vi "Read Last Bus Load.vi"(8 "error in (no error)":errorcluster, 11 "GenBus_Load_Calculator in":refnum<class "CANBus_Load_Calculator.lvclass">) -> (0 "error out":errorcluster, 2 "Bus Load (%)":dbl, 3 "GenBus_Load_Calculator out":refnum<class "CANBus_Load_Calculator.lvclass">)   [LabVIEW 2018, in "NI-XNET Monitor Engine.lvlib" / "XNET-Bus-Load-Calculator.lvlib" / "CANBus_Load_Calculator.lvclass"]
uses:
  CANBus_Load_Calculator.lvclass
  CANBus_Load_Calculator.lvclass/CANBus_Load_Calculator.ctl
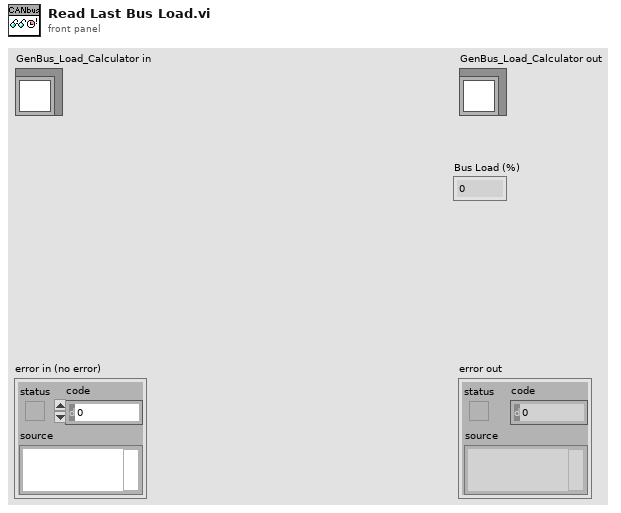
[diagram p1: front panel]
types:
  T1 = typedef "XNET-Bus-Load-Calculator.lvlib/CANBus_Load_Calculator.lvclass/FromCalculator_Data.ctl" = cluster{"Bus Load (%)":dbl}
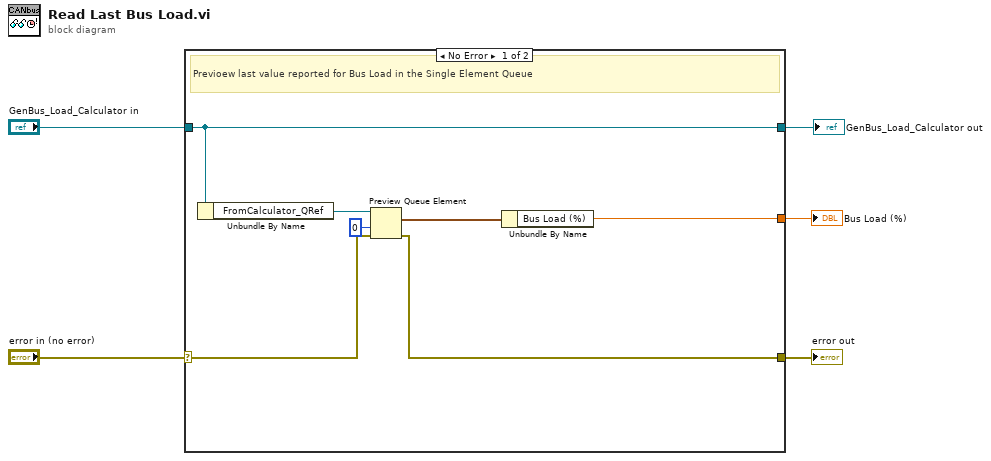
[diagram p0: block diagram]
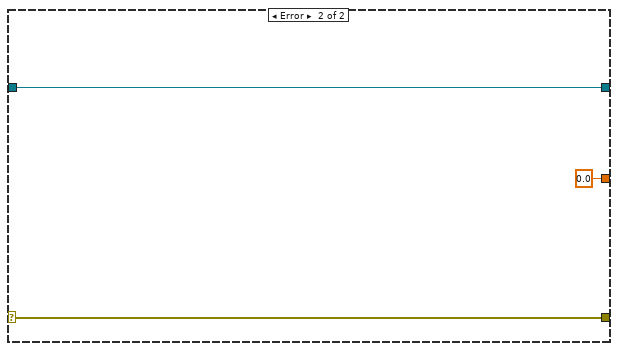
[diagram p2: hidden frame]
diagram:
  n1 = case shown="No Error" "error in (no error)" {
    selector: "error in (no error)" -> [w10 w15]
    tunnel: [w8 w15] -> w4
    tunnel: [w12 w14] -> w1
    tunnel: "GenBus_Load_Calculator in" -> [w12 w14]
    tunnel: [w6 0.0 ("Bus Load (%)")] -> w2
    frame No Error {
      # "Previoew last value reported for Bus Load in the Single Element Queue"
      n2 = Unbundle By Name(w12) -> ("FromCalculator_QRef"=w11:refnum<queue>)
      n3 = Preview Queue Element(queue=w11, timeout in ms (-1)=0, error in (no error)=w10) -> (element=w7:T1, error out=w8:errorcluster)  [unwired: 2 out]
      n4 = Unbundle By Name(w7) -> ("Bus Load (%)"=w6:dbl)
    }
    frame Error {
    }
  }
  "error out" <- w4
  "Bus Load (%)" <- w2
  "GenBus_Load_Calculator out" <- w1
